vi "FGV Werte vorgeben.vi"(6 "Aktion":T1, 9 "D-Filterblock":bool, 11 "P-Flow":bool) -> (1 "D-Filterblock":bool, 3 "P-Flow":bool)   [LabVIEW 2020, in "Regler.lvlib"]
uses:
  Regler.lvlib
  Aktion FGV Werte vorgeben.ctl
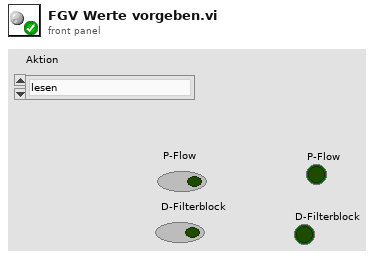
[diagram p1: front panel]
types:
  T1 = typedef "Regler.lvlib/Aktion FGV Werte vorgeben.ctl" = enum16{"lesen", "P-Flow", "D-Filterblock"}
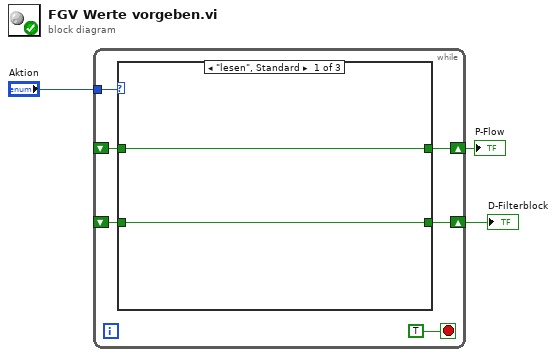
[diagram p0: block diagram]
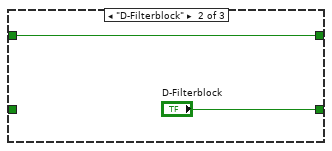
[diagram p2: hidden frame]
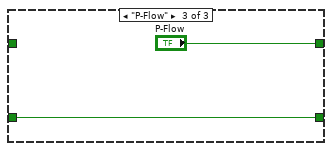
[diagram p3: hidden frame]
diagram:
  n1 = while {
    tunnel: "Aktion" -> [w8]
    shift-right: [w7] -> w2
    shift-left: _ -> [w6]
    shift-right: [w5] -> w1
    shift-left: _ -> [w4]
    stop <- TRUE stop-if-true
    n2 = case shown="\"lesen\", Standard" w8 {
      tunnel: [w11 w13 "P-Flow"] -> w7
      tunnel: w6 -> [w11 w13 _]
      tunnel: [w10 "D-Filterblock" w14] -> w5
      tunnel: w4 -> [w10 _ w14]
      frame "lesen", Default {
      }
      frame "D-Filterblock" {
      }
      frame "P-Flow" {
      }
    }
  }
  "P-Flow" <- w2
  "D-Filterblock" <- w1
